vi "dfd_Dummy_INT MultB.vi"(1 "coef":i16, 2 "x":i16) -> (0 "prod":i32)   [LabVIEW 2017]
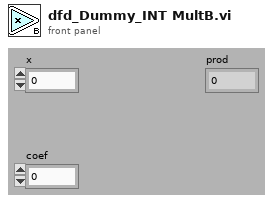
[diagram p1: front panel]
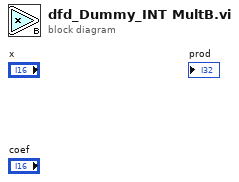
[diagram p0: block diagram]
diagram:
